vi "RX-TX-BPCS-HMI-Modbus.vi"() -> ()   [LabVIEW 2018]
uses:
  <vilib>/Platform/TimedLoop/XDataNode/timing_clust.ctl
  <vilib>/Platform/TimedLoop/XDataNode/nitl_modes.ctl
  <vilib>/Platform/TimedLoop/XDataNode/wakeup.ctl
  <vilib>/Modbus/slave/Create Slave Instance (TCP).vi
  BPCS Global Variables.vi
  <vilib>/Platform/TimedLoop/XDataNode/XDataNode.xnode
  <vilib>/Modbus/slave/Modbus Slave.lvclass
  <vilib>/Platform/TimedLoop/XDataNode/XDNodeRunTimeDep.lvlib
panel:
  out "coil values":bool[](array[boolean])
  out "x":u16[](array[numeric])
  out "*(type *) &x":dbl[](array[numeric])
  in  "Array":dbl[](array[numeric])
  in  "stop":bool
  out "BPCS-SIM-TX-ARRAY":dbl[](array[numeric])
  in  "type 2":u16[](array[numeric])
  out "SIS-BPCS-RX-Array":bool[](array[boolean])
  out "SIM-BPCS-RX-ARRAY":dbl[](array[numeric])
  in  "type":u16[](array[numeric])
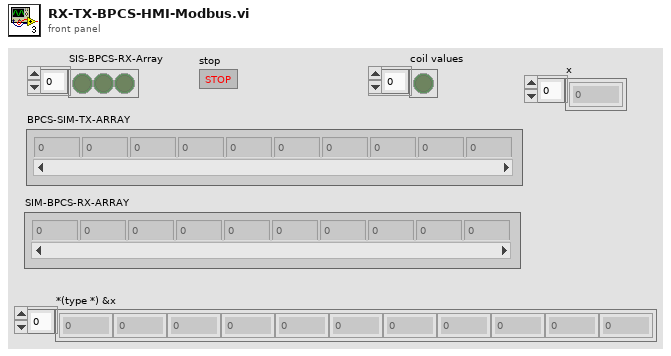
[diagram p1: front panel]
types:
  T1 = typedef "XDNodeRunTimeDep.lvlib/timing_clust.ctl" = cluster{"Expected End [f-1]":u64, "Actual End [f-1]":u64, "Finished Late? [f-1]":bool, "Expected End [i-1]":u64, "Actual End [i-1]":u64, "Finished Late? [i-1]":bool, "Expected Start [i]":u64, "Actual Start [i]":u64, "Expected Start [f]":u64, "Actual Start [f]":u64, "Source Name":string, "Structure Name":string, "Period":i64, "Deadline":i64, "Offset":i64, "Start":i64, "Priority":i32, "Timeout":i32, "Mode":T2, "Wakeup Reason":T3, "Error":errorcluster, "Source Type":string, "Secondary Source Type":string, "Global End Time":u64, "Global Start Time":u64, "Frame Duration":u64, "Iteration Duration":u64, "Assigned CPU":i32, "I/O Scan Engine Mode":u32}
  T2 = typedef "XDNodeRunTimeDep.lvlib/nitl_modes.ctl" = enum32{"No Change", "Process missed periods, maintain original phase", "Discard missed periods, maintain original phase", "Process missed periods, ignore original phase", "Discard missed periods, ignore original phase"}
  T3 = typedef "XDNodeRunTimeDep.lvlib/wakeup.ctl" = enum32{"Normal", "Aborted", "Asynchronous wakeup", "Timing source error", "Timed loop error", "Timeout"}
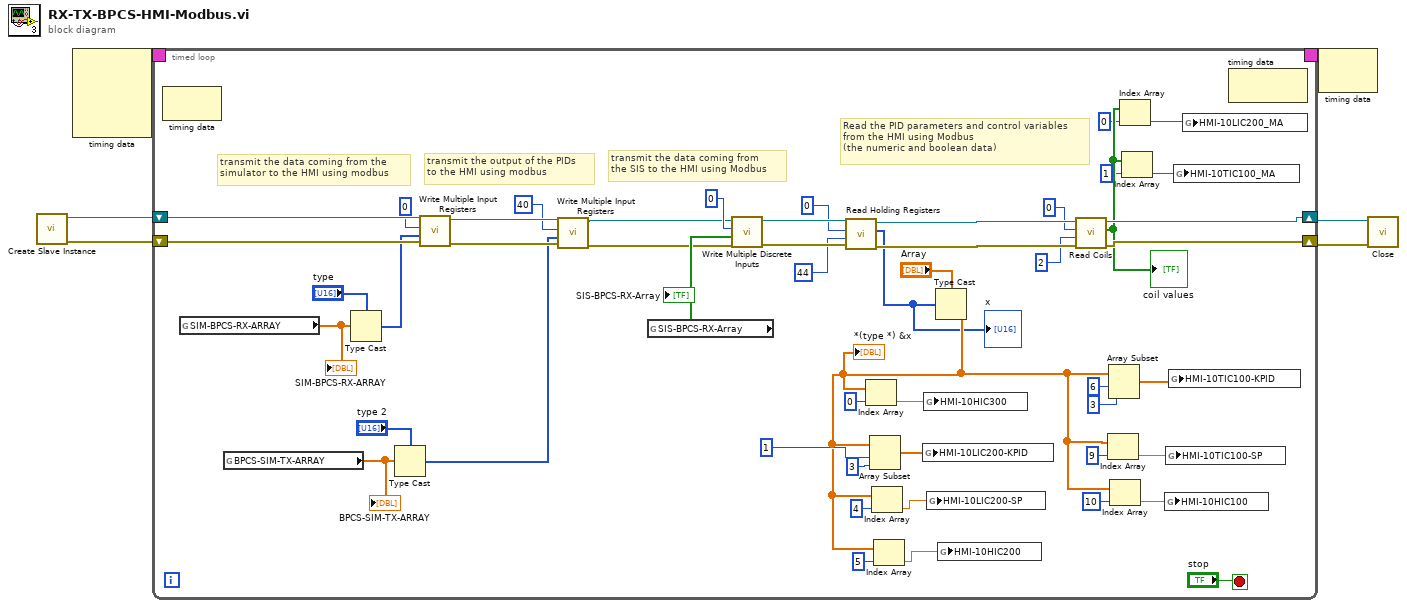
[diagram p0: block diagram]
diagram:
  n1 = call-poly <vilib>:"Create Slave Instance.vi"() -> ("error out"=w3:errorcluster, "TCP slave instance"=w4:refnum<class "Modbus Slave.lvclass">)  [unwired: 10 in]
  n2 = node-c288() -> (w6:T1)  [unwired: 4 in]
  n3 = timed-loop {
    timing: w6 -> [_]
    timing-out: [_] -> w5
    shift-right: [w14] -> w2
    shift-left: w4 -> [w57]
    shift-right: [w13] -> w1
    shift-left: w3 -> [w56]
    stop <- "stop" stop-if-true
    # "Read the PID parameters and control variables \nfrom the HMI using Modbus\n(the numeric and boolean data)"
    # "transmit the data coming from \nthe SIS to the HMI using Modbus"
    # "transmit the output of the PIDs \nto the HMI using modbus"
    # "transmit the data coming from the \nsimulator to the HMI using modbus"
    n4 = node-c288() -> ()  [unwired: 1 in, 1 out]
    n5 = global read "BPCS Global Variables.vi" "SIM-BPCS-RX-ARRAY"() -> (w51:dbl[])
    "SIM-BPCS-RX-ARRAY" <- w51
    n6 = global read "BPCS Global Variables.vi" "BPCS-SIM-TX-ARRAY"() -> (w43:dbl[])
    "BPCS-SIM-TX-ARRAY" <- w43
    n7 = Type Cast(type="type", x=w51) -> (*(type *) &x=w50:u16[])
    n8 = Type Cast(type="type 2", x=w43) -> (*(type *) &x=w42:u16[])
    n9 = call-dynamic "Write Multiple Input Registers.vi"("error in (no error)"=w56, "input register values"=w50, "starting address"=u16 0, "Modbus slave in"=w57) -> ("error out"=w48:errorcluster, "Modbus slave out"=w49:refnum<class "Modbus Slave.lvclass">)  [unwired: 6 in]
    n10 = call-dynamic "Write Multiple Input Registers.vi"("error in (no error)"=w48, "input register values"=w42, "starting address"=u16 40, "Modbus slave in"=w49) -> ("error out"=w46:errorcluster, "Modbus slave out"=w47:refnum<class "Modbus Slave.lvclass">)  [unwired: 6 in]
    n11 = global read "BPCS Global Variables.vi" "SIS-BPCS-RX-Array"() -> (w55:bool[])
    "SIS-BPCS-RX-Array" <- w55
    n12 = call-dynamic "Write Multiple Discrete Inputs.vi"("error in (no error)"=w46, "discrete input values"=w55, "starting address"=u16 0, "Modbus slave in"=w47) -> ("error out"=w39:errorcluster, "Modbus slave out"=w40:refnum<class "Modbus Slave.lvclass">)  [unwired: 6 in]
    n13 = call-dynamic "Read Holding Registers.vi"("error in (no error)"=w39, "number of holding registers"=u16 44, "starting address"=u16 0, "Modbus slave in"=w40) -> ("error out"=w17:errorcluster, "register values"=w7:u16[], "Modbus slave out"=w18:refnum<class "Modbus Slave.lvclass">)  [unwired: 5 in]
    "x" <- w7
    n14 = Type Cast(type="Array", x=w7) -> (*(type *) &x=w22:dbl[])
    "*(type *) &x" <- w22
    n15 = Index Array(array=w22, index=0) -> (element=w34:dbl)
    n16 = Array Subset(array=w22, index=1, length=3) -> (w31:dbl[])
    n17 = Index Array(array=w22, index=4) -> (element=w30:dbl)
    n18 = Index Array(array=w22, index=5) -> (element=w28:dbl)
    n19 = global write "BPCS Global Variables.vi" "HMI-10LIC200-KPID"(w31) -> ()
    n20 = global write "BPCS Global Variables.vi" "HMI-10HIC300"(w34) -> ()
    n21 = global write "BPCS Global Variables.vi" "HMI-10LIC200-SP"(w30) -> ()
    n22 = global write "BPCS Global Variables.vi" "HMI-10HIC200"(w28) -> ()
    n23 = call-dynamic "Read Coils.vi"("error in (no error)"=w17, "number of coils"=u16 2, "starting address"=u16 0, "Modbus slave in"=w18) -> ("error out"=w13:errorcluster, "coil values"=w12:bool[], "Modbus slave out"=w14:refnum<class "Modbus Slave.lvclass">)  [unwired: 5 in]
    "coil values" <- w12
    n24 = Index Array(array=w22, index=9) -> (element=w20:dbl)
    n25 = Array Subset(array=w22, index=6, length=3) -> (w21:dbl[])
    n26 = Index Array(array=w22, index=10) -> (element=w19:dbl)
    n27 = Index Array(array=w12, index=0) -> (element=w9:bool)
    n28 = Index Array(array=w12, index=1) -> (element=w8:bool)
    n29 = global write "BPCS Global Variables.vi" "HMI-10HIC100"(w19) -> ()
    n30 = global write "BPCS Global Variables.vi" "HMI-10TIC100-SP"(w20) -> ()
    n31 = global write "BPCS Global Variables.vi" "HMI-10TIC100-KPID"(w21) -> ()
    n32 = global write "BPCS Global Variables.vi" "HMI-10TIC100_MA"(w8) -> ()
    n33 = global write "BPCS Global Variables.vi" "HMI-10LIC200_MA"(w9) -> ()
    n34 = node-c288() -> ()  [unwired: 1 in, 1 out]
  }
  n35 = node-c288(w5) -> ()  [unwired: 1 out]
  n36 = call-dynamic "Close.vi"("error in (no error)"=w1, "Modbus slave in"=w2) -> ()  [unwired: 9 in, 1 out]
